vi "Queue FGV.vi"(6 "Enum":T2, 8 "error in (no error)":errorcluster, 10 "Modulo a obtener":T1=enum."Error", 11 "Modulos a crear":T1[](array[typedef])) -> (0 "error out":errorcluster, 3 "Queue Ref":refnum<queue>)   [LabVIEW 2018, in "Mensajes.lvlib"]
uses:
  Mensajes.lvlib
  Controles/FGV Opciones.ctl
  Controles/Lista Modulos.ctl
  Controles/Mensaje Data.ctl
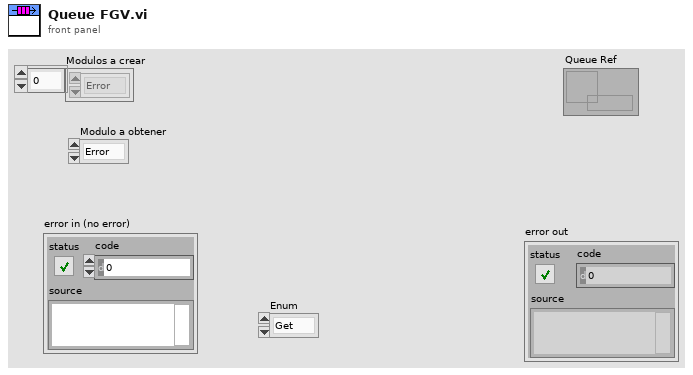
[diagram p1: front panel]
types:
  T1 = typedef "Lista Modulos.ctl" = enum16{"Math", "Error", "Front", "Database", "Nuevos items"}
  T2 = typedef "FGV Opciones.ctl" = enum16{"Get", "Create", "Destroy"}
  T3 = typedef "Mensaje Data.ctl" = cluster{"Mensaje":string, "Dato":variant}
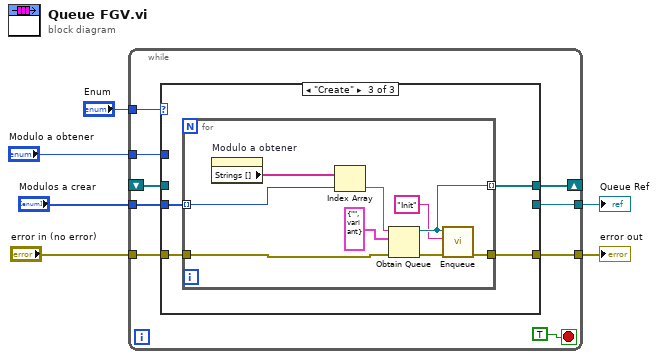
[diagram p0: block diagram]
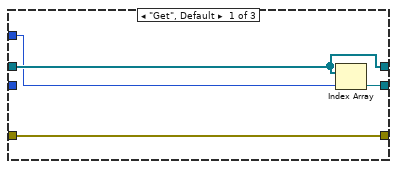
[diagram p2: hidden frame]
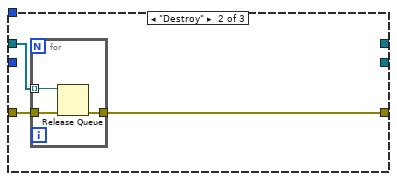
[diagram p3: hidden frame]
diagram:
  n1 = while {
    tunnel: "Enum" -> [w14]
    tunnel: "Modulos a crear" -> [w13]
    tunnel: "error in (no error)" -> [w12]
    tunnel: [w11] -> w3
    shift-right: [w10] -> _
    shift-left: _ -> [w9]
    tunnel: "Modulo a obtener" -> [w8]
    tunnel: [w7] -> w1
    stop <- TRUE stop-if-true
    n2 = case shown="\"Create\"" w14 {
      tunnel: w13 -> [_ _ w29]
      tunnel: w12 -> [w16 w21 w28]
      tunnel: [w16 w20 w27] -> w11
      tunnel: [w19 _ w26] -> w10
      tunnel: w9 -> [w19 w22 _]
      tunnel: w8 -> [w18 _ _]
      tunnel: [w17 _ _] -> w7
      frame "Get", Default {
        n3 = Index Array(array=w19, index=w18) -> (element=w17:refnum<queue>)
      }
      frame "Destroy" {
        n4 = for {
          tunnel: w22 -> [w25] mode=indexing
          tunnel: w21 -> [w24]
          tunnel: [w23] -> w20
          n5 = Release Queue(queue=w25, error in (no error)=w24) -> (error out=w23:errorcluster)  [unwired: 1 in, 2 out]
        }
      }
      frame "Create" {
        n6 = for {
          tunnel: w29 -> [w37] mode=indexing
          tunnel: w28 -> [w35]
          tunnel: [w31] -> w27
          tunnel: [w33] -> w26 mode=indexing
          n7 = property on="Modulo a obtener" class="Enum (strict)"() -> ("Strings []"=w38:string[])  [unwired: 2 in, 2 out]
          n8 = Index Array(array=w38, index=w37) -> (element=w36:string)
          n9 = Obtain Queue(name (unnamed)=w36, element data type=T3 {"Mensaje"="", "Dato"=variant} ("Cluster"), error in (no error)=w35) -> (queue out=w33:refnum<queue>, error out=w32:errorcluster)  [unwired: 2 in, 1 out]
          n10 = call "Enqueue.vi"("error in (no error)"=w32, "Mensaje"="Init", "Queue in"=w33) -> ("error out"=w31:errorcluster)  [unwired: 8 in]
        }
      }
    }
  }
  "error out" <- w3
  "Queue Ref" <- w1
